vi "testCreateTcpIpConnectionServersAandB.vi"(8 "error in":errorcluster) -> (0 "error out":errorcluster)   [LabVIEW 2018]
uses:
  <vilib>/addons/_JKI Toolkits/Caraya/classes/Assert/Assert True.vi
  src/TcpServer/TcpServer.lvclass
  <vilib>/addons/_JKI Toolkits/Caraya/classes/Test/Test.lvclass
  <vilib>/addons/_JKI Toolkits/Caraya/classes/Assert/Assert.lvclass
panel:
  out "Run Server B error":errorcluster
  out "Run Server A error":errorcluster
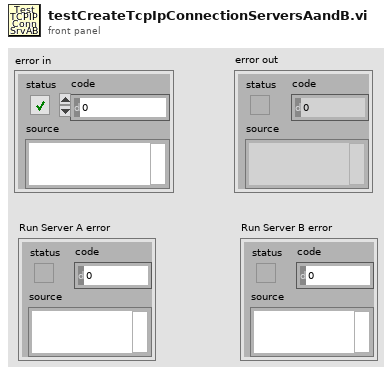
[diagram p1: front panel]
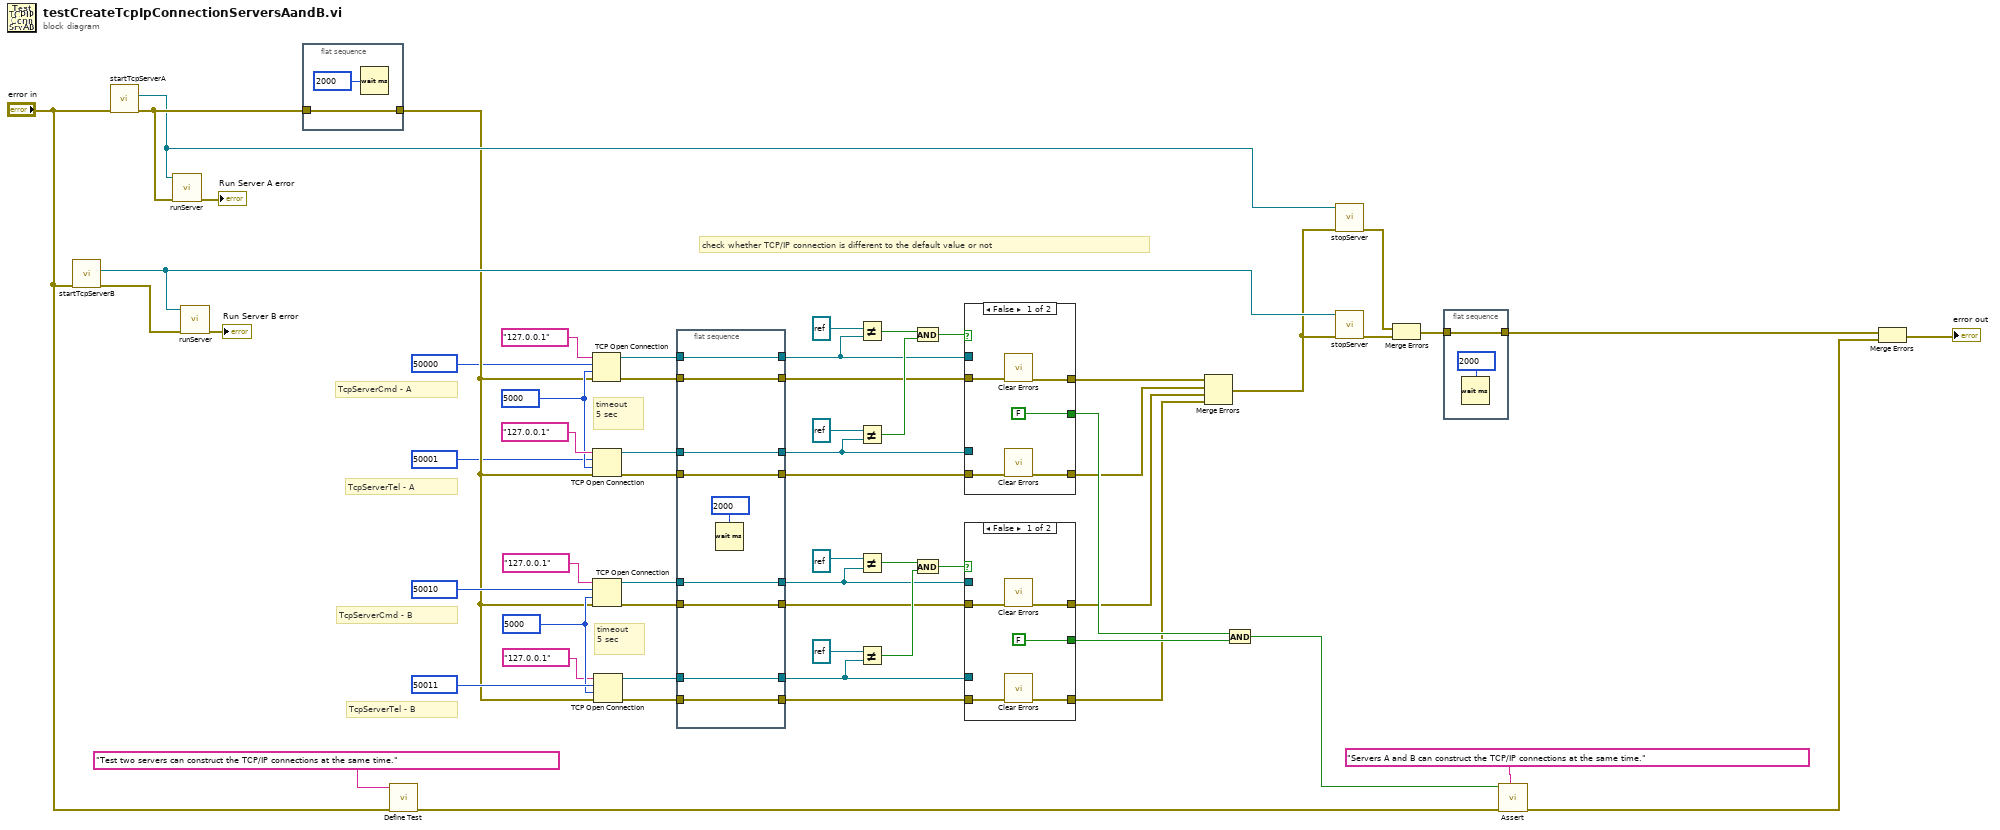
[diagram p0: block diagram]
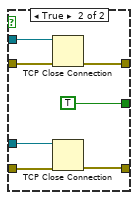
[diagram p2: hidden frame]
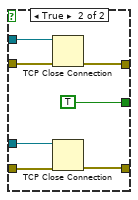
[diagram p3: hidden frame]
diagram:
  w8 = 5000 ("timeout ms (60000)")
  w41 = 5000 ("timeout ms (60000)")
  # "timeout\n5 sec"
  # "timeout\n5 sec"
  # "check whether TCP/IP connection is different to the default value or not"
  # "TcpServerTel - B"
  # "TcpServerCmd - B"
  # "TcpServerTel - A"
  # "TcpServerCmd - A"
  n1 = call "startTcpServerB.vi"("error in (no error)"="error in") -> ("error out"=w52:errorcluster, "TcpServer out"=w24:refnum<class "TcpServer.lvclass">)  [unwired: 8 in, 1 out]
  n2 = call "startTcpServerA.vi"("error in (no error)"="error in") -> ("error out"=w59:errorcluster, "TcpServer out"=w58:refnum<class "TcpServer.lvclass">)  [unwired: 8 in, 1 out]
  n3 = call "runServer.vi"("error in (no error)"=w59, "TcpServer in"=w58) -> ("error out (no error)"=→"Run Server A error":errorcluster)  [unwired: 8 in, 1 out]
  n4 = call "runServer.vi"("error in (no error)"=w52, "TcpServer in"=w24) -> ("error out (no error)"=→"Run Server B error":errorcluster)  [unwired: 8 in, 1 out]
  n5 = flat-sequence {
    tunnel: w59 -> [w62]
    tunnel: [w62] -> w7
    frame #0 {
      n6 = Wait (ms)(milliseconds to wait=u32 2000) -> ()  [unwired: 1 out]
    }
  }
  n7 = call <vilib>:"Define Test.vi"("error in (no error)"="error in", "Label (VI Title)"="Test two servers can construct the TCP/IP connections at the same time.") -> ("error out"=w55:errorcluster)  [unwired: 9 in]
  n8 = TCP Open Connection(address="127.0.0.1", remote port or service name=u16 50000, timeout ms (60000)=w8, error in (no error)=w7) -> (connection ID=w4:refnum<k5>, error out=w3:errorcluster)  [unwired: 1 in]
  n9 = TCP Open Connection(address="127.0.0.1", remote port or service name=u16 50001, timeout ms (60000)=w8, error in (no error)=w7) -> (connection ID=w2:refnum<k5>, error out=w1:errorcluster)  [unwired: 1 in]
  n10 = TCP Open Connection(address="127.0.0.1", remote port or service name=u16 50010, timeout ms (60000)=w41, error in (no error)=w7) -> (connection ID=w31:refnum<k5>, error out=w29:errorcluster)  [unwired: 1 in]
  n11 = TCP Open Connection(address="127.0.0.1", remote port or service name=u16 50011, timeout ms (60000)=w41, error in (no error)=w7) -> (connection ID=w27:refnum<k5>, error out=w25:errorcluster)  [unwired: 1 in]
  n12 = flat-sequence {
    tunnel: [w72] -> w36
    tunnel: w4 -> [w72]
    tunnel: [w71] -> w35
    tunnel: w3 -> [w71]
    tunnel: [w70] -> w34
    tunnel: w2 -> [w70]
    tunnel: [w69] -> w33
    tunnel: w1 -> [w69]
    tunnel: [w68] -> w32
    tunnel: w31 -> [w68]
    tunnel: [w67] -> w30
    tunnel: w29 -> [w67]
    tunnel: [w66] -> w28
    tunnel: w27 -> [w66]
    tunnel: [w65] -> w26
    tunnel: w25 -> [w65]
    frame #0 {
      n13 = Wait (ms)(milliseconds to wait=u32 2000) -> ()  [unwired: 1 out]
    }
  }
  n14 = Not Equal?(x=refnum<k5> refnum ("connection ID"), y=w36) -> (x != y?=w45:bool)
  n15 = Not Equal?(x=refnum<k5> refnum ("connection ID"), y=w34) -> (x != y?=w44:bool)
  n16 = Not Equal?(x=refnum<k5> refnum ("connection ID"), y=w32) -> (x != y?=w43:bool)
  n17 = Not Equal?(x=refnum<k5> refnum ("connection ID"), y=w28) -> (x != y?=w42:bool)
  n18 = Compound Arithmetic op=AND(w45, w44) -> (w38:bool)
  n19 = Compound Arithmetic op=AND(w43, w42) -> (w37:bool)
  n20 = case shown="False" w38 {
    tunnel: w36 -> [_ w84]
    tunnel: w34 -> [_ w83]
    tunnel: w33 -> [w76 w82]
    tunnel: w35 -> [w77 w81]
    tunnel: [FALSE TRUE] -> w23
    tunnel: [w74 w79] -> w20
    tunnel: [w73 w78] -> w19
    frame False {
      n21 = call <vilib>:"Clear Errors.vi"("error in (no error)"=w77) -> ("error out"=w74:errorcluster)  [unwired: 5 in, 1 out]
      n22 = call <vilib>:"Clear Errors.vi"("error in (no error)"=w76) -> ("error out"=w73:errorcluster)  [unwired: 5 in, 1 out]
    }
    frame True {
      n23 = TCP Close Connection(connection ID=w84, error in (no error)=w81) -> (error out=w79:errorcluster)  [unwired: 1 in, 1 out]
      n24 = TCP Close Connection(connection ID=w83, error in (no error)=w82) -> (error out=w78:errorcluster)  [unwired: 1 in, 1 out]
    }
  }
  n25 = case shown="False" w37 {
    tunnel: w32 -> [_ w96]
    tunnel: w28 -> [_ w95]
    tunnel: w26 -> [w88 w94]
    tunnel: w30 -> [w89 w93]
    tunnel: [FALSE TRUE] -> w22
    tunnel: [w86 w91] -> w18
    tunnel: [w85 w90] -> w17
    frame False {
      n26 = call <vilib>:"Clear Errors.vi"("error in (no error)"=w89) -> ("error out"=w86:errorcluster)  [unwired: 5 in, 1 out]
      n27 = call <vilib>:"Clear Errors.vi"("error in (no error)"=w88) -> ("error out"=w85:errorcluster)  [unwired: 5 in, 1 out]
    }
    frame True {
      n28 = TCP Close Connection(connection ID=w96, error in (no error)=w93) -> (error out=w91:errorcluster)  [unwired: 1 in, 1 out]
      n29 = TCP Close Connection(connection ID=w95, error in (no error)=w94) -> (error out=w90:errorcluster)  [unwired: 1 in, 1 out]
    }
  }
  n30 = Merge Errors(w20, w19, w18, w17) -> (w16:errorcluster)
  n31 = Compound Arithmetic op=AND(w23, w22) -> (w21:bool)
  n32 = call "stopServer.vi"("error in (no error)"=w16, "tcpServer in"=w58) -> ("error out"=w15:errorcluster)  [unwired: 8 in, 1 out]
  n33 = call "stopServer.vi"("error in (no error)"=w16, "tcpServer in"=w24) -> ("error out"=w14:errorcluster)  [unwired: 8 in, 1 out]
  n34 = Merge Errors(w15, w14) -> (w13:errorcluster)
  n35 = flat-sequence {
    tunnel: w13 -> [w97]
    tunnel: [w97] -> w12
    frame #0 {
      n36 = Wait (ms)(milliseconds to wait=u32 2000) -> ()  [unwired: 1 out]
    }
  }
  n37 = call-poly <vilib>:"Assert.vi"("Label"="Servers A and B can construct the TCP/IP connections at the same time.", "error in (no error)"=w55, "True?"=w21) -> ("error out"=w11:errorcluster)  [unwired: 8 in]
  n38 = Merge Errors(w12, w11) -> (→"error out":errorcluster)
